vi "AddChannel(Force).vi"(8 "error in (no error)":errorcluster, 10 "T560Channel.lvclass":refnum<class "T560Channel.lvclass">, 11 "T560Session in":refnum<class "T560Session.lvclass">) -> (0 "error out":errorcluster, 3 "T560Session out":refnum<class "T560Session.lvclass">)   [LabVIEW 2020, in "T560Session.lvclass"]
uses:
  T560Session.lvclass
  T560Channel.lvclass
  T560Session.lvclass/T560Session.ctl
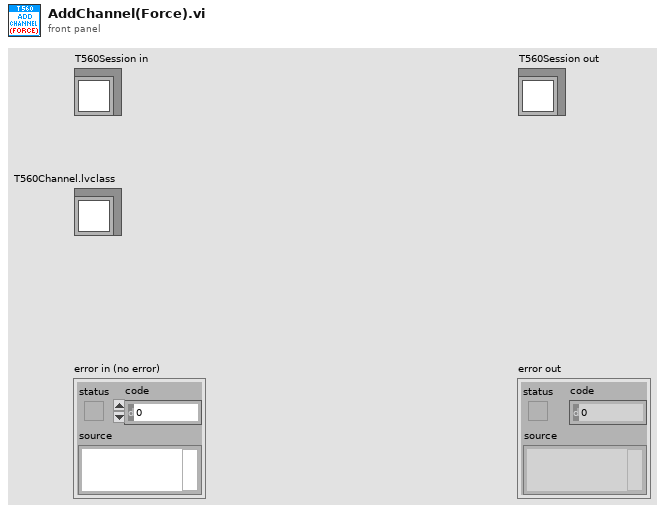
[diagram p1: front panel]
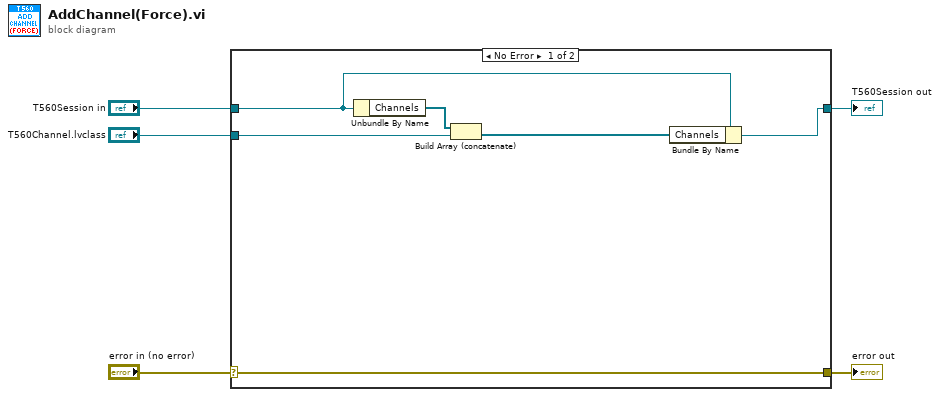
[diagram p0: block diagram]
diagram:
  n1 = case shown="No Error" "error in (no error)" {
    selector: "error in (no error)" -> [w11 w13]
    tunnel: [w11 w13] -> w4
    tunnel: [w9 w12] -> w2
    tunnel: "T560Session in" -> [w10 w12]
    tunnel: "T560Channel.lvclass" -> [w7 _]
    frame No Error {
      n2 = Unbundle By Name(w10) -> ("Channels"=w8:refnum<class "T560Channel.lvclass">[])
      n3 = Build Array (concatenate)(w8, w7) -> (w6:refnum<class "T560Channel.lvclass">[])
      n4 = Bundle By Name(cluster=w10, "Channels"=w6) -> (w9:refnum<class "T560Session.lvclass">)
    }
    frame Error {
    }
  }
  "error out" <- w4
  "T560Session out" <- w2
